vi "UpdateDashboardDisplay.vi"() -> (3 "Team Dashboard Data":T1)   [LabVIEW 2012]
uses:
  Robot Global Data.vi
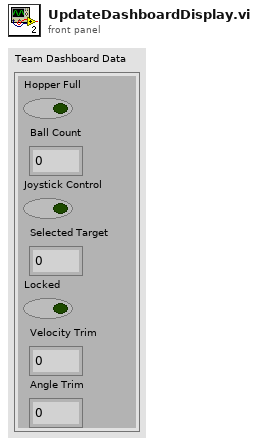
[diagram p1: front panel]
types:
  T1 = cluster{"Hopper Full":bool, "Ball Count":dbl, "Joystick Control":bool, "Selected Target":dbl, "Locked":bool, "Velocity Trim":dbl, "Angle Trim":dbl}
  T2 = cluster{"Position":cluster{"X":dbl, "Y":dbl}, "Distance (ft)":dbl}[]
  T3 = cluster{"Position":cluster{"X":dbl, "Y":dbl}, "Distance (ft)":dbl}
  T4 = cluster{"Hopper Full":bool, "Ball Count":dbl, "Joystick Control":bool, "Selected Target":i32, bool, "Velocity Trim":dbl, "Angle Trim":dbl}
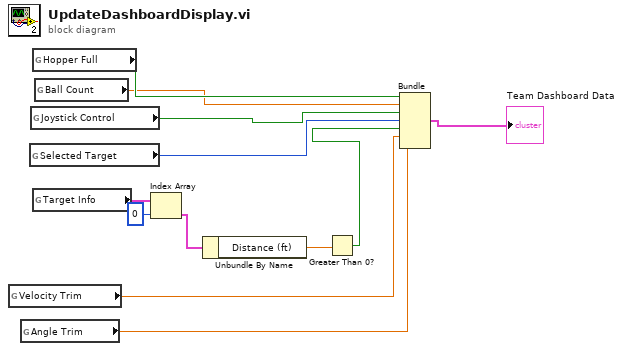
[diagram p0: block diagram]
diagram:
  n1 = global read "Robot Global Data.vi" "Velocity Trim"() -> (w2:dbl)
  n2 = global read "Robot Global Data.vi" "Angle Trim"() -> (w1:dbl)
  n3 = global read "Robot Global Data.vi" "Selected Target"() -> (w9:i32)
  n4 = global read "Robot Global Data.vi" "Joystick Control"() -> (w10:bool)
  n5 = global read "Robot Global Data.vi" "Hopper Full"() -> (w12:bool)
  n6 = global read "Robot Global Data.vi" "Target Info"() -> (w8:T2)
  n7 = global read "Robot Global Data.vi" "Ball Count"() -> (w11:dbl)
  n8 = Index Array(array=w8, index=0) -> (element=w6:T3)
  n9 = Unbundle By Name(w6) -> ("Distance (ft)"=w5:dbl)
  n10 = Greater Than 0?(x=w5) -> (x > 0?=w4:bool)
  n11 = Bundle("Hopper Full"=w12, "Ball Count"=w11, "Joystick Control"=w10, "Selected Target"=w9, w4, "Velocity Trim"=w2, "Angle Trim"=w1) -> (→"Team Dashboard Data":T4)  [unwired: 1 in]
